vi "CAD@SetRobotTool__Parameter.vi"(1 "ParamterIn":string) -> (0 "ParamterOut":string)   [LabVIEW 2019]
panel:
  in  "ToolName":string(combo)
  in  "RobotName":string(combo)
  in  "Confirm":bool
  # "CAD@SetRobotTool $Robott,$TooltName"
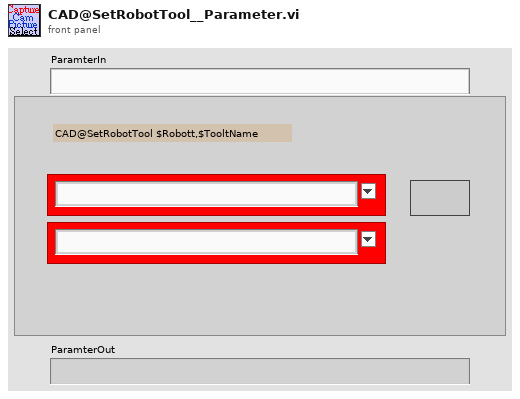
[diagram p1: front panel]
types:
  T1 = enum16{"Init", "Load Tool", "Load Part", "Get Tool Property", "Get Part Property", "Set Tool to End Matrix", "Set Part to Tool Matrix", "Calculate Part to Tool & End Matrix", "Create Part From Copy", "Delete Part"}
  T2 = cluster{"Tool Name":string[], "Part Name":string[]}
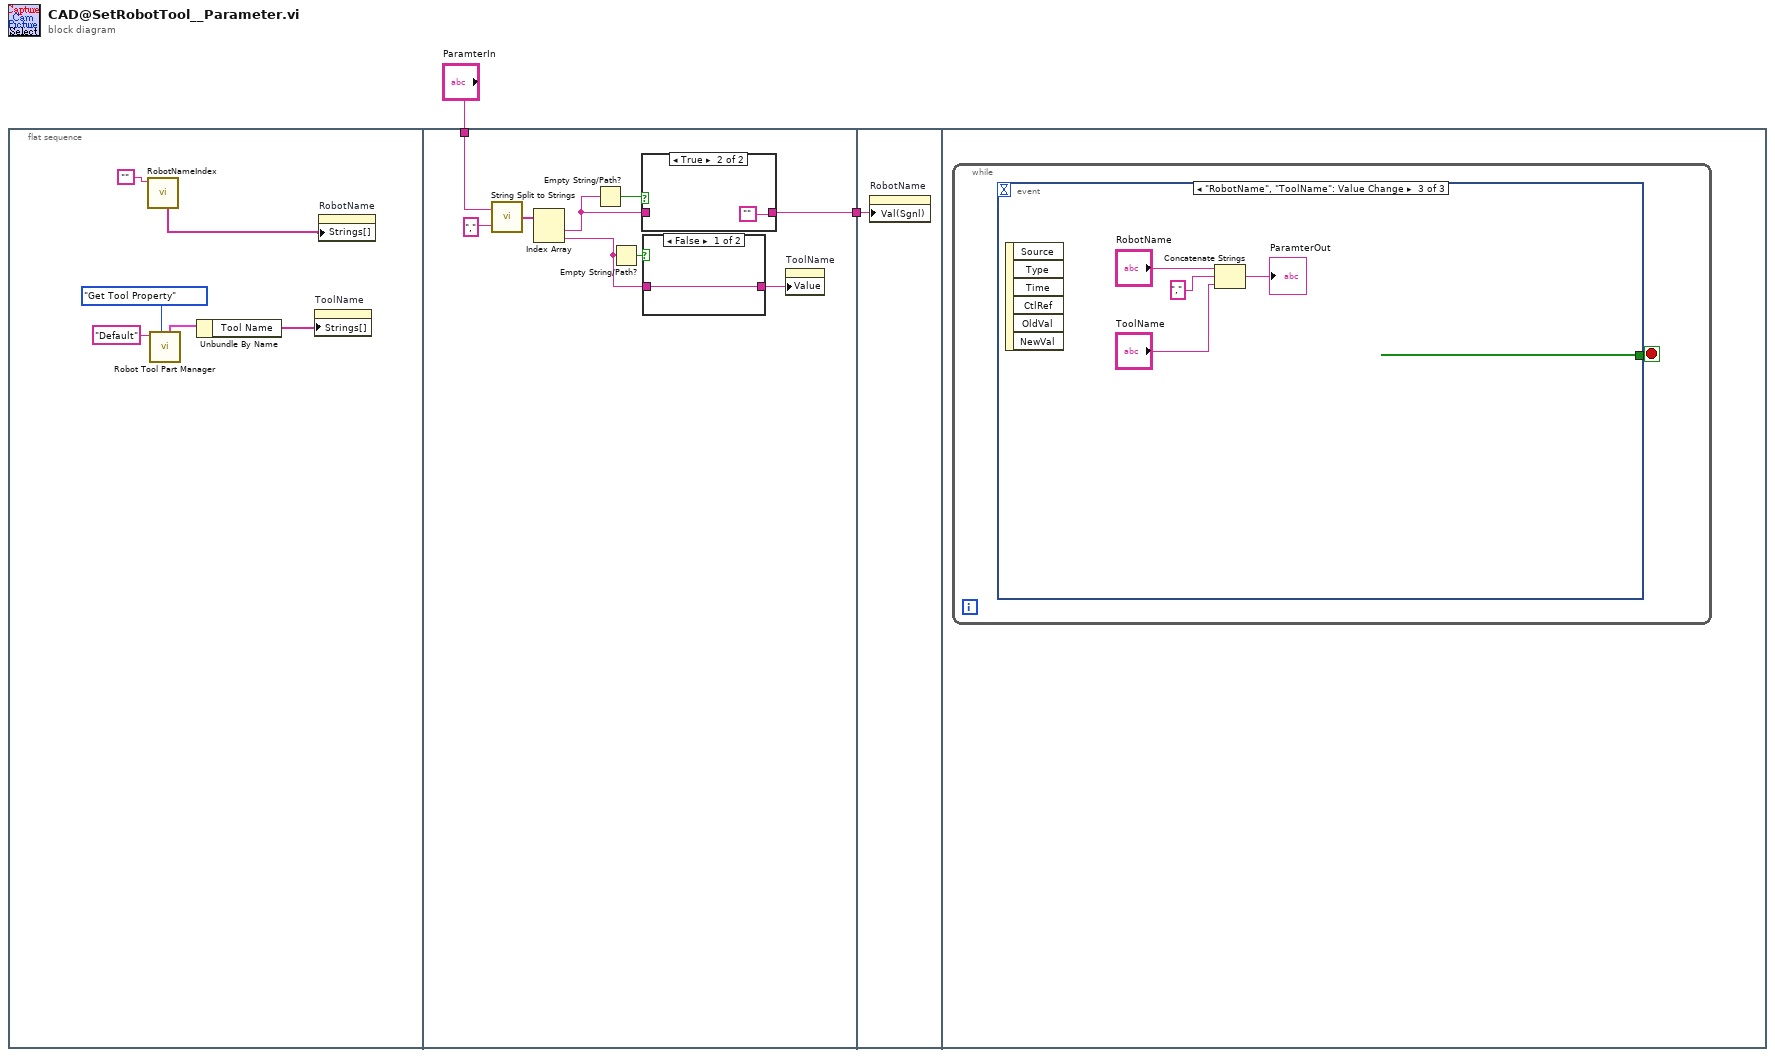
[diagram p0: block diagram]
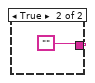
[diagram p2: hidden frame]
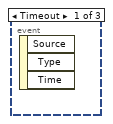
[diagram p4: hidden frame]
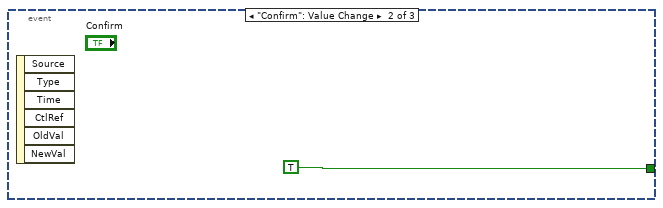
[diagram p5: hidden frame]
diagram:
  n1 = flat-sequence {
    tunnel: "ParamterIn" -> [w15]
    tunnel: [w10] -> w1
    tunnel: w1 -> [w22]
    frame #0 {
      n2 = call "RobotNameIndex.vi"("RobotName"="") -> ("RobotNameList"=w3:string[])  [unwired: 8 in, 2 out]
      n3 = call "Robot Tool Part Manager.vi"("CMD"=T1."Get Tool Property", "Tool / Part Name"="Default") -> ("NameList"=w6:T2)  [unwired: 4 in, 5 out]
      n4 = Unbundle By Name(w6) -> ("Tool Name"=w5:string[])
      n5 = property on="ToolName" class="CmbBox"("Strings[]"=w5) -> ()  [unwired: 2 in, 2 out]
      n6 = property on="RobotName" class="CmbBox"("Strings[]"=w3) -> ()  [unwired: 2 in, 2 out]
    }
    frame #1 {
      n7 = call "String Split to Strings.vi"("search string/char (-)"=",", "String"=w15) -> ("Array"=w17:string[])
      n8 = Index Array(array=w17) -> (element #1=w11:string, element #2=w12:string)  [unwired: 2 in]
      n9 = Empty String/Path?(string/path=w11) -> (empty?=w14:bool)
      n10 = Empty String/Path?(string/path=w12) -> (empty?=w13:bool)
      n11 = case shown="True" w14 {
        tunnel: w11 -> [w20 _]
        tunnel: [w20 ""] -> w10
        frame False {
        }
        frame True {
        }
      }
      n12 = case shown="False" w13 {
        tunnel: [w18 ""] -> w9
        tunnel: w12 -> [w18 _]
        frame False {
        }
        frame True {
        }
      }
      n13 = property on="ToolName" class="CmbBox"("Value"=w9) -> ()  [unwired: 2 in, 2 out]
    }
    frame #2 {
      n14 = property on="RobotName" class="CmbBox"("Val(Sgnl)"=w22) -> ()  [unwired: 2 in, 2 out]
    }
    frame #3 {
      n15 = while {
        stop <- w23 stop-if-true
        n16 = event shown="[2] \"RobotName\", \"ToolName\": Value Change" {
          selector: _ -> [_ _ _]
          dyn-events: _ -> [_ _ _]
          timeout: _ -> [_ _ _]
          tunnel: [_ TRUE _] -> w23
          event Timeout {
            n17 = event-data() -> ()  [unwired: 1 in, 3 out]
          }
          event "Confirm": Value Change {
            n18 = event-data() -> ()  [unwired: 1 in, 6 out]
          }
          event "RobotName", "ToolName": Value Change {
            n19 = event-data() -> ()  [unwired: 1 in, 6 out]
            n20 = Concatenate Strings("RobotName", "," ("element"), "ToolName") -> (→"ParamterOut":string)
          }
        }
      }
    }
  }
